vi "Create.vi"(10 "Config Element":refnum<class "Config Element.lvclass">) -> (3 "ConfigElementValue out":refnum<class "ConfigElementValue.lvclass">)   [LabVIEW 2020, in "Volatus.lvlib" / "ConfigElementValue.lvclass"]
uses:
  ConfigElementValue.lvclass
  ConfigElementValue.lvclass/ConfigElementValue.ctl
  lv-cdm/CDM-Config/Config Element/Config Element.lvclass
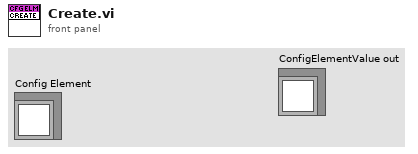
[diagram p1: front panel]
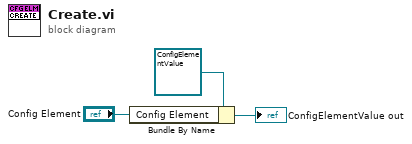
[diagram p0: block diagram]
diagram:
  n1 = Bundle By Name(cluster=refnum<class "ConfigElementValue.lvclass"> refnum ("ConfigElementValue in"), "Config Element"="Config Element") -> (→"ConfigElementValue out":refnum<class "ConfigElementValue.lvclass">)
